vi "C37EvtParamsErrors.vi"(8 "error in (no error)":errorcluster, 10 "dblSignalParams in":dbl[][](array[numeric])) -> (0 "error out":errorcluster, 2 "dblSignalParams out":dbl[][](array[numeric]))   [LabVIEW 2017, in "EventPlugins.lvlib" / "C37EvtPlugin.lvclass"]
uses:
  C37EvtPlugin.lvclass
  <vilib>/Utility/error.llb/Error Cluster From Error Code.vi
  <vilib>/ErrorRing/Error Ring.xnode
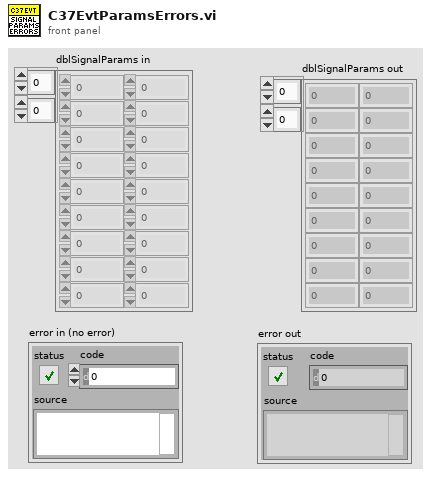
[diagram p1: front panel]
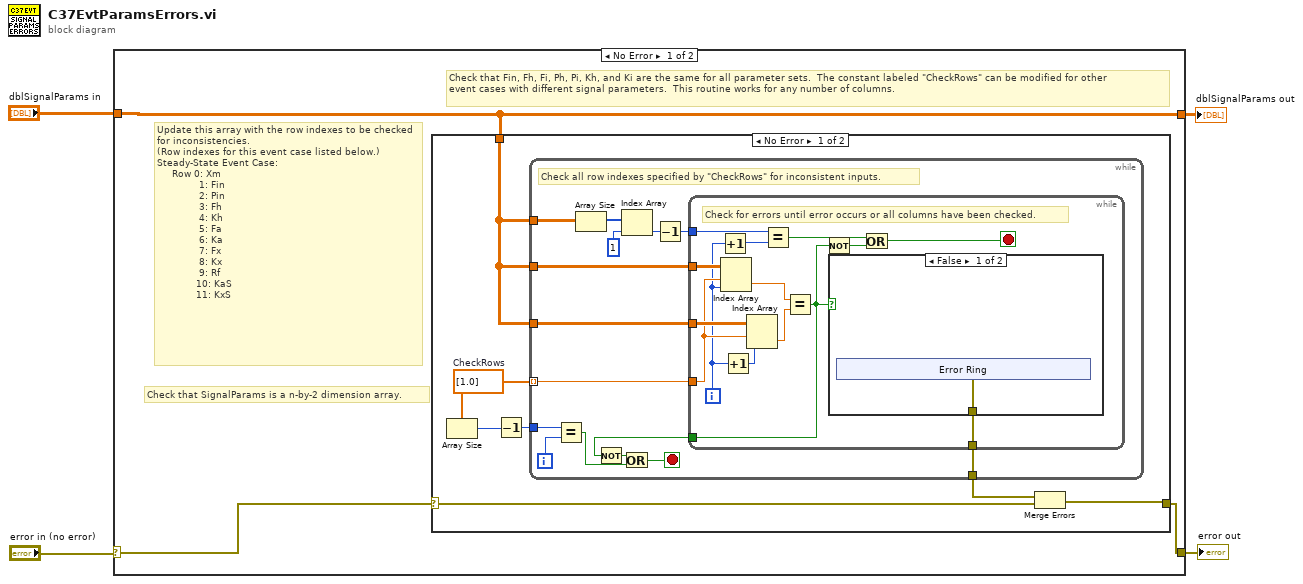
[diagram p0: block diagram]
diagram:
  n1 = case shown="No Error" "error in (no error)" {
    selector: "error in (no error)" -> [w5 w52]
    tunnel: [w6 w52] -> w3
    tunnel: "dblSignalParams in" -> [w7 w51]
    tunnel: [w7 w51] -> w1
    frame No Error {
      # "Update this array with the row indexes to be checked for inconsistencies.  \n(Row indexes for this event case listed below.)\nSteady-State Event Case:\n     Row 0: Xm\n              1: Fin\n              2: Pin\n              3: Fh\n              4: Kh\n              5: Fa\n              6: Ka\n              7: Fx\n              8: Kx\n              9: Rf\n             10: KaS\n             11: KxS"
      # "Check that Fin, Fh, Fi, Ph, Pi, Kh, and Ki are the same for all parameter sets.  The constant labeled \"CheckRows\" can be modified for other\nevent cases with different signal parameters.  This routine works for any number of columns."
      # "Check that SignalParams is a n-by-2 dimension array."
      n2 = case shown="No Error" w5 {
        selector: w5 -> [w8 w50]
        tunnel: w7 -> [w14 _]
        tunnel: [w10 w50] -> w6
        frame No Error {
          w13 = dbl[] [1.0]  # CheckRows
          n3 = Array Size(array=w13) -> (size(s)=w11:i32)
          n4 = Decrement(x=w11) -> (x-1=w12:i32)
          n5 = while {
            tunnel: w14 -> [w29]
            tunnel: w14 -> [w28]
            tunnel: w14 -> [w25]
            tunnel: w13 -> [w24] mode=indexing
            tunnel: w12 -> [w21]
            tunnel: [w16] -> w9
            i -> [w20]
            stop <- w19 stop-if-true
            # "Check all row indexes specified by \"CheckRows\" for inconsistent inputs."
            n6 = Equal?(x=w21, y=w20) -> (x = y?=w17:bool)
            n7 = Array Size(array=w25) -> (size(s)=w27:i32[])
            n8 = Index Array(array=w27, index=1) -> (element=w23:i32)
            n9 = Decrement(x=w23) -> (x-1=w22:i32)
            n10 = while {
              tunnel: w29 -> [w43]
              tunnel: w28 -> [w42]
              tunnel: w24 -> [w40]
              tunnel: w22 -> [w34]
              tunnel: [w31] -> w18
              tunnel: [w30] -> w16
              i -> [w35]
              stop <- w37 stop-if-true
              # "Check for errors until error occurs or all columns have been checked."
              n11 = Increment(x=w35) -> (x+1=w32:i32)
              n12 = Index Array(array=w43, index (row)=w40, index (col)=w35) -> (element=w38:dbl)
              n13 = Increment(x=w35) -> (x+1=w41:i32)
              n14 = Index Array(array=w42, index (row)=w40, index (col)=w41) -> (element=w39:dbl)
              n15 = Equal?(x=w34, y=w32) -> (x = y?=w36:bool)
              n16 = Equal?(x=w38, y=w39) -> (x = y?=w31:bool)
              n17 = Not(x=w31) -> (.not. x?=w33:bool)
              n18 = case shown="False" w31 {
                tunnel: [w44 _] -> w30
                frame False {
                  n19 = xnode "Error Ring"() -> ("error out"=w44:errorcluster)
                }
                frame True {
                }
              }
              n20 = Or(x=w36, y=w33) -> (x .or. y?=w37:bool)
            }
            n21 = Not(x=w18) -> (.not. x?=w15:bool)
            n22 = Or(x=w15, y=w17) -> (x .or. y?=w19:bool)
          }
          n23 = Merge Errors(w9, w8) -> (w10:errorcluster)
        }
        frame Error {
        }
      }
    }
    frame Error {
    }
  }
  "dblSignalParams out" <- w1
  "error out" <- w3
